vi "SetCheckedStatus.vi"(8 "error in (no error)":errorcluster, 9 "Checked":bool, 10 "MenuItem":refnum<class "MGI_MenuItem.lvclass">, 11 "VI":refnum<class "MGI_VI.lvclass">) -> (0 "error out":errorcluster, 3 "VI":refnum<class "MGI_VI.lvclass">)   [LabVIEW 2016, in "MGI_VI.lvclass"]
doc: "Sets the clicked status of the menu item.\n\nAuthored by Derek E. Trepanier\nsupport@mooregoodideas.com\nwww.mooregoodideas.com\n\nCopyright (c) 2012, Moore Good Ideas, Inc.\n\nAll rights reserved.\n\nRedistribution and use in source and binary forms, with or without modification, are permitted provided that the following conditions are met:\n\n * Redistributions of source code must retain the above copyright notice, this list of conditions and the following disclaimer.\n * Redistributions in binary form must reproduce the above copyright notice, this list of conditions and the following disclaimer in the documentation and/or other materials provided with the distribution.\n * Neither the name of Moore Good Ideas, Inc. nor the names of its contributors may be used to endorse or promote products derived from this software without specific prior written permission.\n\nTHIS SOFTWARE IS PROVIDED BY THE COPYRIGHT HOLDERS AND CONTRIBUTORS \"AS IS\" AND ANY EXPRESS OR IMPLIED WARRANTIES, INCLUDING, BUT NOT LIMITED TO, THE IMPLIED WARRANTIES OF MERCHANTABILITY AND FITNESS FOR A PARTICULAR PURPOSE ARE DISCLAIMED. IN NO EVENT SHALL THE COPYRIGHT OWNER OR CONTRIBUTORS BE LIABLE FOR ANY DIRECT, INDIRECT, INCIDENTAL, SPECIAL, EXEMPLARY, OR CONSEQUENTIAL DAMAGES (INCLUDING, BUT NOT LIMITED TO, PROCUREMENT OF SUBSTITUTE GOODS OR SERVICES; LOSS OF USE, DATA, OR PROFITS; OR BUSINESS INTERRUPTION) HOWEVER CAUSED AND ON ANY THEORY OF LIABILITY, WHETHER IN CONTRACT, STRICT LIABILITY, OR TORT (INCLUDING NEGLIGENCE OR OTHERWISE) ARISING IN ANY WAY OUT OF THE USE OF THIS SOFTWARE, EVEN IF ADVISED OF THE POSSIBILITY OF SUCH DAMAGE."
uses:
  <userlib>/_MGI/Menu Building/MenuTypes/Vi/MGI_VI.lvclass
  <userlib>/_MGI/Menu Building/MenuItem/MGI_MenuItem.lvclass
  <userlib>/_MGI/Menu Building/MenuTypes/Vi/MGI_VI.lvclass/MGI_VI.ctl
  <userlib>/_MGI/Menu Building/MenuItem/Read Full Tag.vi
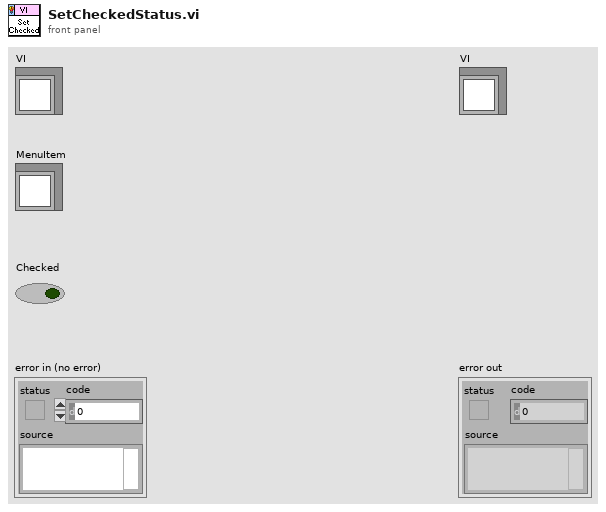
[diagram p1: front panel]
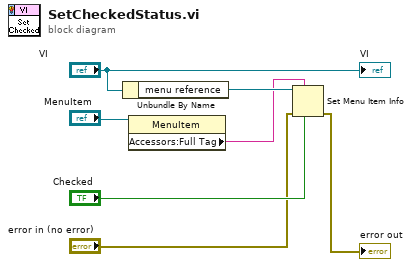
[diagram p0: block diagram]
diagram:
  n1 = Unbundle By Name("VI") -> ("menu reference"=w5:refnum<k9>)
  n2 = property class="MenuItem"(reference="MenuItem") -> ("Accessors:Full Tag"=w4:string)  [unwired: 1 in, 2 out]
  n3 = Set Menu Item Info(6:"Checked", 7:w4, 8:"error in (no error)", 11:w5) -> (0:→"error out":errorcluster)  [unwired: 3 in, 1 out]
  "VI" <- "VI"
